vi "Calibration.vi"   [LabVIEW 2012]
uses:
  Global Variables.vi
  Global Refnums.vi
types:
  T1 = typedef "WPI_AnalogChannelDevRef.ctl" = cluster{"DevStatus":errorcluster, "Analog Module":T2, "Analog Channel":T3}
  T2 = typedef "FPGA_TypedefAnalogModule.ctl" = enum16{"Analog Module 1", "Analog Module 2"}
  T3 = typedef "FPGA_AIChannel.ctl" = enum8{"AI 1", "AI 2", "AI 3", "AI 4", "AI 5", "AI 6", "AI 7", "AI 8", "Invalid"}
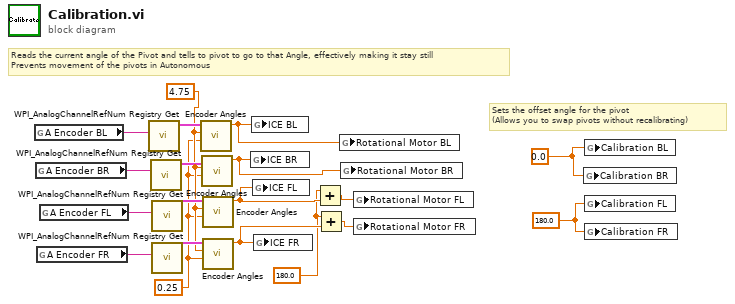
[diagram p0: block diagram]
diagram:
  w1 = 180.0
  w12 = 0.25
  w13 = 4.75
  w18 = 0.0
  w19 = 180.0
  # "Sets the offset angle for the pivot\n(Allows you to swap pivots without recalibrating)"
  # "Reads the current angle of the Pivot and tells to pivot to go to that Angle, effectively making it stay still\nPrevents movement of the pivots in Autonomous"
  n1 = global read "Global Refnums.vi" "A Encoder BL"() -> (w11:string)
  n2 = global read "Global Refnums.vi" "A Encoder BR"() -> (w10:string)
  n3 = global read "Global Refnums.vi" "A Encoder FR"() -> (w8:string)
  n4 = global read "Global Refnums.vi" "A Encoder FL"() -> (w9:string)
  n5 = call <vilib>:"WPI_AnalogChannelRefNum Registry Get.vi"("refnum name"=w11) -> ("AIDeviceRef"=w17:T1)  [unwired: 9 in, 1 out]
  n6 = call <vilib>:"WPI_AnalogChannelRefNum Registry Get.vi"("refnum name"=w10) -> ("AIDeviceRef"=w16:T1)  [unwired: 9 in, 1 out]
  n7 = call <vilib>:"WPI_AnalogChannelRefNum Registry Get.vi"("refnum name"=w9) -> ("AIDeviceRef"=w15:T1)  [unwired: 9 in, 1 out]
  n8 = call <vilib>:"WPI_AnalogChannelRefNum Registry Get.vi"("refnum name"=w8) -> ("AIDeviceRef"=w14:T1)  [unwired: 9 in, 1 out]
  n9 = call "Encoder Angles.vi"("Bottom Voltage"=w12, "Top Voltage"=w13, "AIDeviceRef Encoder"=w17) -> ("Encoder Angle"=w6:dbl)  [unwired: 8 in]
  n10 = call "Encoder Angles.vi"("Bottom Voltage"=w12, "Top Voltage"=w13, "AIDeviceRef Encoder"=w16) -> ("Encoder Angle"=w5:dbl)  [unwired: 8 in]
  n11 = call "Encoder Angles.vi"("Bottom Voltage"=w12, "Top Voltage"=w13, "AIDeviceRef Encoder"=w15) -> ("Encoder Angle"=w7:dbl)  [unwired: 8 in]
  n12 = call "Encoder Angles.vi"("Bottom Voltage"=w12, "Top Voltage"=w13, "AIDeviceRef Encoder"=w14) -> ("Encoder Angle"=w4:dbl)  [unwired: 8 in]
  n13 = global write "Global Variables.vi" "ICE BR"(w5) -> ()
  n14 = global write "Global Variables.vi" "ICE BL"(w6) -> ()
  n15 = global write "Global Variables.vi" "ICE FL"(w7) -> ()
  n16 = global write "Global Variables.vi" "ICE FR"(w4) -> ()
  n17 = Add(x=w1, y=w7) -> (x+y=w3:dbl)
  n18 = Add(x=w1, y=w4) -> (x+y=w2:dbl)
  n19 = global write "Global Variables.vi" "Rotational Motor BL"(w6) -> ()
  n20 = global write "Global Variables.vi" "Rotational Motor BR"(w5) -> ()
  n21 = global write "Global Variables.vi" "Rotational Motor FL"(w3) -> ()
  n22 = global write "Global Variables.vi" "Rotational Motor FR"(w2) -> ()
  n23 = global write "Global Variables.vi" "Calibration BR"(w18) -> ()
  n24 = global write "Global Variables.vi" "Calibration BL"(w18) -> ()
  n25 = global write "Global Variables.vi" "Calibration FL"(w19) -> ()
  n26 = global write "Global Variables.vi" "Calibration FR"(w19) -> ()
